vi "New Panel Reference Receive.vi"(8 "error in (no error)":errorcluster, 9 "VI Refnum":refnum<vi>, 10 "Label":string, 11 "Microscope in":refnum<class "Microscope.lvclass">) -> (0 "error out":errorcluster, 3 "Microscope out":refnum<class "Microscope.lvclass">)   [LabVIEW 2020]
uses:
  Microscope Controller Messages/InsertPanel Msg/InsertPanel Msg.lvclass
  Microscope.lvclass
  E:/Development/DevHardSoftware/MMicroscopyAF/Model/HAL Layer/Device/Device/Device.lvclass
  C:/Program Files/National Instruments/LabVIEW 2020/vi.lib/ActorFramework/Actor/Actor.lvclass
  E:/Development/DevHardSoftware/MMicroscopyAF/Model/HAL Layer/Microscope/Microscope/Microscope.lvclass
  E:/Development/DevHardSoftware/MMicroscopyAF/Communication/Communication.lvclass
  <vilib>/ActorFramework/Message Enqueuer/Message Enqueuer.lvclass
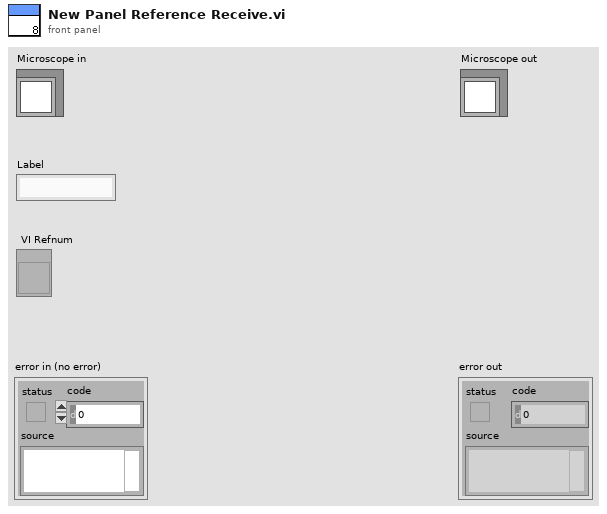
[diagram p1: front panel]
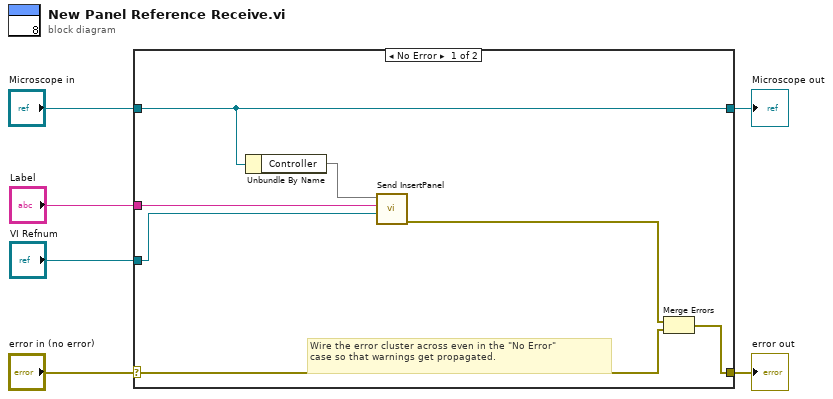
[diagram p0: block diagram]
diagram:
  n1 = case shown="No Error" "error in (no error)" {
    selector: "error in (no error)" -> [w9 w15]
    tunnel: [w8 w15] -> w5
    tunnel: [w13 w14] -> w3
    tunnel: "Microscope in" -> [w13 w14]
    tunnel: "Label" -> [w11 _]
    tunnel: "VI Refnum" -> [w10 _]
    frame No Error {
      # "Wire the error cluster across even in the \"No Error\"\ncase so that warnings get propagated."
      n2 = Unbundle By Name(w13) -> ("Controller"=w12)
      n3 = call "Send InsertPanel.vi"("VI Refnum"=w10, "Device Type"=w11, "Message Enqueuer"=w12) -> ("error out"=w7:errorcluster)  [unwired: 7 in, 1 out]
      n4 = Merge Errors(w7, w9) -> (w8:errorcluster)
    }
    frame Error {
    }
  }
  "error out" <- w5
  "Microscope out" <- w3
